vi "Decode FPGA Packet.vi"(10 "Array":u8[](array[numeric])) -> (2 "xml string":string)   [LabVIEW 2014]
uses:
  FPGA Telemetry.ctl
  Vehicle Status/Subsystem Status.ctl
  Vehicle Status/Subsystem Status Severity.ctl
  Vehicle Status/Subsystem Status Message.ctl
  AIR Status.ctl
  Reason for Shutdown.ctl
  Dash LED Status.ctl
  FPGA/SPI v2/ADXL345 Output.ctl
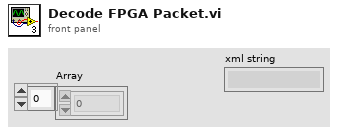
[diagram p1: front panel]
types:
  T1 = typedef "FPGA Telemetry.ctl" = cluster{"CPU Load":cluster{"Total (%)":dbl, "Time Critical (%)":dbl, "Timed Structures (%)":dbl, "High (%)":dbl, "Above Normal (%)":dbl, "Normal (%)":dbl, "Background (%)":dbl, "Idle (%)":dbl, "ISR (%)":dbl}, "SVehicleStatus":cluster{"BMS Status":T2, "MC Status":T2, "Shutdown Status":T2, "sbRIO Status":T2, "Vehicle Status":T2, "Shutdown State":enum16{"NI.SC.Initial", "NI.SC.History", "NI.SC.ShallowHistory", "NI.SC.Terminal", "Coolant Pump Started/AIR's On", "AIRs On", "Precharge", "TSMS Off"}, "AIR Status":T5, "Remote Return to Pits":bool, "Reason for Shutdown":T6, "MC State Machine Status":enum16{"NI.SC.Initial", "NI.SC.History", "NI.SC.ShallowHistory", "NI.SC.Terminal", "Broadcast Diag", "Let Current Drop then Disable AIR's", "Enabled", "Disabled"}}, "iPhone HF Data":cluster{"gXiPhone":dbl, "gYiPhone":dbl, "gZiPhone":dbl, "nYawXiPhone":dbl, "nYawYiPhone":dbl, "nYawZiPhone":dbl}, "iPhone LF Data":cluster{"nLatiPhone":dbl, "nLongiPhone":dbl, "nGPSiPhone":dbl}, "stop":bool, "VSupplyOffset":fxp<+,12,4>, "VsbRIOSupply":fxp<+/-,25,6>, "bFPGALED":bool, "TSBRIO":fxp<+/-,33,17>, "rTPS2Unscaled":fxp<+/-,16,1>, "rTPS1Unscaled":fxp<+/-,16,1>, "bTPSConsistent":bool, "bTPSInRange":bool, "rThrottle":fxp<+/-,33,22>, "VTPS2":fxp<+/-,24,5>, "rTPS2":fxp<+/-,31,22>, "VTPS1":fxp<+/-,24,5>, "rTPS1":fxp<+/-,31,22>, "rTPS2Max":fxp<+,16,4>, "rTPS2Min":fxp<+,16,4>, "rTPS1Max":fxp<+,16,4>, "rTPS1Min":fxp<+,16,4>, "bCoolantPumpEnable":bool, "bRTDSEnable":bool, "bTSMSInStatus":bool, "bPosAIREnable":bool, "bBMSOK":bool, "bIMDOK":bool, "bBSPDOK":bool, "bSBRIOOK2":bool, "bSBRIOOK1":bool, "bTSMSOutStatus":bool, "eGreenDash":T7, "eYellowDash":T7, "eRedDash":T7, "bMotorControllerEnable":bool, "tCurrentLap":u32, "bNewLap":bool, "tLastLap":u32, "tLapMin":u32, "V5VSupply":fxp<+/-,24,5>, "bWheelRL":bool, "bWheelRR":bool, "bWheelFR":bool, "bWheelFL":bool, "VBrakePressureR":fxp<+/-,24,5>, "VBrakePressureF":fxp<+/-,24,5>, "bWheelRRStopped":bool, "bWheelRLStopped":bool, "bWheelFRStopped":bool, "bWheelFLStopped":bool, "tWheelRLPeriod":u32, "tWheelRRPeriod":u32, "tWheelFRPeriod":u32, "tWheelFLPeriod":u32, "bBrakeLight":bool, "VShockRR":fxp<+/-,24,5>, "VShockRL":fxp<+/-,24,5>, "VShockFR":fxp<+/-,24,5>, "VShockFL":fxp<+/-,24,5>, "IHighCurrent":fxp<+/-,24,15>, "ILowCurrent":fxp<+/-,24,15>, "pBrakeR":fxp<+,26,13>, "pBrakeF":fxp<+,26,13>, "bHighCurrentOK":bool, "bLowCurrentOK":bool, "bBrakeROK":bool, "bBrakeFOK":bool, "VSteerWheelMiddle":fxp<+/-,26,5>, "aSteerWheel":fxp<+/-,31,13>, "nWheelFL":fxp<+/-,32,16>, "nWheelFR":fxp<+/-,32,16>, "nWheelRL":fxp<+/-,32,16>, "nWheelRR":fxp<+/-,32,16>, "ADXL345 Output":T8, "Tire Diameter(m)":fxp<+,16,1>, "vWheelRR":fxp<+/-,32,18>, "vWheelRL":fxp<+/-,32,18>, "vWheelFR":fxp<+/-,32,18>, "vWheelFL":fxp<+/-,32,18>, "vWheelLowest":fxp<+/-,32,18>, "vWheelHighest":fxp<+/-,32,18>, "bAccel":bool, "vAxleF":fxp<+/-,33,19>, "vCar":fxp<+/-,33,19>, "sLap":fxp<+,32,12>, "rSlipRL":fxp<+/-,12,1>, "rSlipRR":fxp<+/-,12,1>, "rSlipFL":fxp<+/-,12,1>, "rSlipFR":fxp<+/-,12,1>, "NLap":u8, "tLapReference":u32, "tFastestLap":u32}
  T2 = typedef "Subsystem Status.ctl" = cluster{"eStatusSeverity":T3, "NValue":sgl, "CMessage":T4, "bNotOK":bool}
  T3 = typedef "Subsystem Status Severity.ctl" = enum16{"Okay", "Short Warning", "Long Warning", "Return to Pits", "Error", "Danger"}
  T4 = typedef "Subsystem Status Message.ctl" = enum16{"ControllerTemperature", "MotorTemperature", "BatteryTemperature", "BatteryLowVoltage", "LVBattery", "sbRIOTemperature", "Precharge", "BSPD", "IMD", "RemoteReturnToPits", "EStopInterrupted", "NoCellComms", "MCOverSpeed", "MCOverCurrent", "MCOverVoltage", "MCInverterOverTemp", "MCDirectionCommand", "MCInverterTimeout", "MCDesatFault", "MCHWOverCurrent", "MCUnderVoltage", "MCCommandMessageLost", "MotorOverTemp", "MCModAOverTemp", "MCModBOverTemp", "MCModCOverTemp", "MCPCBOverTemp", "MCGateDrv1OverTemp", "MCDateDrv2OverTemp", "MCCurrentSensorFault", "MCResolverNotConnected", "ShutdownLatchTripped", "UnknownBMS", "RemoteEmergency"}
  T5 = typedef "AIR Status.ctl" = enum16{"Off", "Precharge", "On"}
  T6 = typedef "Reason for Shutdown.ctl" = enum16{"None", "BMS", "Shutdown", "sbRIO", "MC", "Remote"}
  T7 = typedef "Dash LED Status.ctl" = enum16{"Off", "Flashing", "On"}
  T8 = typedef "ADXL345 Output.ctl" = cluster{"X":fxp<+/-,14,4>, "Y":fxp<+/-,14,4>, "Z":fxp<+/-,14,4>}
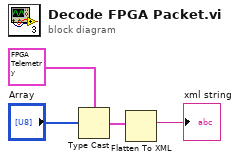
[diagram p0: block diagram]
diagram:
  n1 = Type Cast(type=T1 {"CPU Load"={"Total (%)"=0.0, "Time Critical (%)"=0.0, "Timed Structures (%)"=0.0, "High (%)"=0.0, "Above Normal (%)"=0.0, "Normal (%)"=0.0, "Background (%)"=0.0, "Idle (%)"=0.0, "ISR (%)"=0.0}, "SVehicleStatus"={"BMS Status"={"eStatusSeverity"=enum."Okay", "NValue"=0.0, "CMessage"=enum."ControllerTemperature", "bNotOK"=FALSE}, "MC Status"={"eStatusSeverity"=enum."Okay", "NValue"=0.0, "CMessage"=enum."ControllerTemperature", "bNotOK"=FALSE}, "Shutdown Status"={"eStatusSeverity"=enum."Okay", "NValue"=0.0, "CMessage"=enum."ControllerTemperature", "bNotOK"=FALSE}, "sbRIO Status"={"eStatusSeverity"=enum."Okay", "NValue"=0.0, "CMessage"=enum."ControllerTemperature", "bNotOK"=FALSE}, "Vehicle Status"={"eStatusSeverity"=enum."Okay", "NValue"=0.0, "CMessage"=enum."ControllerTemperature", "bNotOK"=FALSE}, "Shutdown State"=enum."NI.SC.Initial", "AIR Status"=enum."Off", "Remote Return to Pits"=FALSE, "Reason for Shutdown"=enum."None", "MC State Machine Status"=enum."NI.SC.Initial"}, "iPhone HF Data"={"gXiPhone"=0.0, "gYiPhone"=0.0, "gZiPhone"=0.0, "nYawXiPhone"=0.0, "nYawYiPhone"=0.0, "nYawZiPhone"=0.0}, "iPhone LF Data"={"nLatiPhone"=0.0, "nLongiPhone"=0.0, "nGPSiPhone"=0.0}, "stop"=FALSE, "VSupplyOffset"=8.890625, "VsbRIOSupply"=13.101043701171875, "bFPGALED"=FALSE, "TSBRIO"=27.25, "rTPS2Unscaled"=0.0, "rTPS1Unscaled"=0.0, "bTPSConsistent"=FALSE, "bTPSInRange"=FALSE, "rThrottle"=0.0, "VTPS2"=1.0001773834228516, "rTPS2"=0.0, "VTPS1"=3.619058609008789, "rTPS1"=0.0, "rTPS2Max"=0.27001953125, "rTPS2Min"=0.489990234375, "rTPS1Max"=0.6201171875, "rTPS1Min"=0.41015625, "bCoolantPumpEnable"=FALSE, "bRTDSEnable"=FALSE, "bTSMSInStatus"=FALSE, "bPosAIREnable"=FALSE, "bBMSOK"=FALSE, "bIMDOK"=FALSE, "bBSPDOK"=FALSE, "bSBRIOOK2"=FALSE, "bSBRIOOK1"=FALSE, "bTSMSOutStatus"=FALSE, "eGreenDash"=enum."Off", "eYellowDash"=enum."Off", "eRedDash"=enum."Off", "bMotorControllerEnable"=FALSE, "tCurrentLap"=0, "bNewLap"=TRUE, "tLastLap"=0, "tLapMin"=0, "V5VSupply"=0.0, "bWheelRL"=FALSE, "bWheelRR"=FALSE, "bWheelFR"=FALSE, "bWheelFL"=FALSE, "VBrakePressureR"=0.4820976257324219, "VBrakePressureF"=0.4808177947998047, "bWheelRRStopped"=TRUE, "bWheelRLStopped"=TRUE, "bWheelFRStopped"=TRUE, "bWheelFLStopped"=TRUE, "tWheelRLPeriod"=0, "tWheelRRPeriod"=0, "tWheelFRPeriod"=0, "tWheelFLPeriod"=0, "bBrakeLight"=TRUE, "VShockRR"=0.3793773651123047, "VShockRL"=0.3444976806640625, "VShockFR"=0.3425788879394531, "VShockFL"=0.3892974853515625, "IHighCurrent"=-20.724609375, "ILowCurrent"=4.353515625, "pBrakeR"=0.0, "pBrakeF"=0.0, "bHighCurrentOK"=FALSE, "bLowCurrentOK"=FALSE, "bBrakeROK"=FALSE, "bBrakeFOK"=FALSE, "VSteerWheelMiddle"=0.34827280044555664, "aSteerWheel"=124.90449142456055, "nWheelFL"=0.0, "nWheelFR"=0.0, "nWheelRL"=0.0, "nWheelRR"=0.0, "ADXL345 Output"={"X"=0.0, "Y"=0.0, "Z"=0.0}, "Tire Diameter(m)"=0.0, "vWheelRR"=0.0, "vWheelRL"=0.0, "vWheelFR"=0.0, "vWheelFL"=0.0, "vWheelLowest"=0.0, "vWheelHighest"=0.0, "bAccel"=FALSE, "vAxleF"=0.0, "vCar"=0.0, "sLap"=0.0, "rSlipRL"=0.0, "rSlipRR"=0.0, "rSlipFL"=0.0, "rSlipFR"=0.0, "NLap"=0, "tLapReference"=0, "tFastestLap"=0} ("FPGA Telemetry"), x="Array") -> (*(type *) &x=w2:T1)
  n2 = Flatten To XML(anything=w2) -> (xml string=→"xml string":string)
